vi "Settings.vi"() -> ()   [LabVIEW 2023]
uses:
  <vilib>/userDefined/High Color/nirio_resource_hc.ctl
panel:
  in  "?":T1(tab)
  in  "Current follower 1\n (AI-3)":dbl(ring)=-1e-08 items=["Raw"=1.0, "1mA (Ivium Compactstat.h)"=-0.001, "100uA (ivium Compactstat.h)"=-0.0001, "1uA (Ivium Compactstat.h)"=-1e-06, "100nA (Ivium Compactstat.h)"=-1e-07, "10nA (Ivium Compactstat.h)"=-1e-08, "1nA (Ivium Compactstat.h)"=-1e-09, "100pA (Ivium Compactstat.h)"=-1e-10, "10pA (Ivium Compactstat.h)"=-1e-11, "100 uA/V"=0.0001, "10 uA/V"=1e-05, "1 uA/V"=1e-06, "100 nA/V"=1e-07, "10 nA/V (0.1 mV/pA)"=1e-08, "0.2 mV/pA"=5e-09, "0.5 mV/pA"=2e-09, "1 nA/V (1 mV/pA)"=1e-09, "2 mV/pA"=5e-10, "5 mV/pA"=2e-10, "100 pA/V (10 mV/pA)"=1e-10, "20 mV/pA"=5e-11, "10 pA/V"=1e-11, "1 pA/V"=1e-12, "100 fA/V"=1e-13, "10 fA/V"=1e-14, "1 fA/V"=1e-15]
  in  "Current follower 3\n(AI-6)":dbl(ring)=1e-09 items=["Raw"=1.0, "100 uA/V"=0.0001, "10 uA/V"=1e-05, "1 uA/V"=1e-06, "100 nA/V"=1e-07, "10 nA/V (0.1 mV/pA)"=1e-08, "0.2 mV/pA"=5e-09, "0.5 mV/pA"=2e-09, "1 nA/V (1 mV/pA)"=1e-09, "2 mV/pA"=5e-10, "5 mV/pA"=2e-10, "100 pA/V (10 mV/pA)"=1e-10, "20 mV/pA"=5e-11, "10 pA/V"=1e-11, "1 pA/V"=1e-12, "100 fA/V"=1e-13, "10 fA/V"=1e-14, "1 fA/V"=1e-15]
  in  "Current follower 2 \n(AI-4)":dbl(ring)=-1.0 items=["Raw (Ivium Compactstat.h)"=-1.0, "10uA (Ivium Compactstat.h)"=-1e-05, "1uA (Ivium Compactstat.h)"=-1e-06, "100nA (Ivium Compactstat.h)"=-1e-07, "10nA (Ivium Compactsta.h)"=-1e-08, "1nA (Ivium Compactstat.h)"=-1e-09, "100pA (Ivium Compactstat.h)"=-1e-10, "10pA (Ivium Compactstat.h)"=-1e-11, "Raw"=1.0, "100 uA/V"=0.0001, "10 uA/V"=1e-05, "1 uA/V"=1e-06, "100 nA/V"=1e-07, "10 nA/V (0.1 mV/pA)"=1e-08, "0.2 mV/pA"=5e-09, "0.5 mV/pA"=2e-09, "1 nA/V (1 mV/pA)"=1e-09, "2 mV/pA"=5e-10, "5 mV/pA"=2e-10, "100 pA/V (10 mV/pA)"=1e-10, "20 mV/pA"=5e-11, "10 pA/V"=1e-11, "1 pA/V"=1e-12, "100 fA/V"=1e-13, "10 fA/V"=1e-14, "1 fA/V"=1e-15]
  in  "Lock In Sensitivity":dbl(ring)=1.0 items=["1V/V"=1.0, "500mV/V"=0.5, "200mV/V"=0.2]
  in  "Expand":dbl(ring)=100.0 items=["100"=100.0, "10"=10.0, "1"=1.0]
  in  "Percentage Offset":dbl min=0.0 max=100.0 step=0.0001 format="%#.12e"
  in  "Current follower for AC?":u8(ring) items=["C1", "C2", "C3"]
  in  "Sample Time (µs)":u32=4 min=2
  in  "Samples per Data Point":u16(ring)=512 items=["1"=1, "2"=2, "4"=4, "8"=8, "16"=16, "32"=32, "64"=64, "128"=128, "256"=256, "512"=512, "1024"=1024, "2048"=2048, "4096"=4096, "8192"=8192]
  in  "Save Folder Path":path=path "Z:/"
  in  "TempFilePath":path=path "C:/GitHub/WEC-SPM_Temp/test.tdms"
  in  "channel names":string[](array[string])=["X (um)", "Y (um)", "Z (um)", "V1 (V)", "V2 (V)", "Current1 (A)", "Current 2 (A)", "Current 3 (A)", "FeedbackType ", "Line Number", "Lockin Amplitude", "Lockin  Phase", "dt(s)"]
  in  "FPGA Target Device":T2="RIO0" caption="RIO Device"
  in  "Command Voltage2 Ratio 2":dbl(ring)=5.0 items=["1:1"=1.0, "5:1"=5.0, "10:1"=10.0]
  in  "Z piezo maximum range (µm)":dbl=200.0
  in  "Y piezo maximum range (µm)":dbl=200.0
  in  "X piezo maximum range (µm)":dbl=200.0
  in  "Command Voltage Ratio":dbl(ring)=1.0 items=["1:1"=1.0, "5:1"=5.0, "10:1"=10.0]
  out "Z (-10 to 10V)":bool
  out "X (-10 to 10V)":bool
  out "Y (-10 to 10V)":bool
  out "FPGA Speed [Hz]":i64=40000000
  in  "Host Path":path=path "C:/GitHub/WEC-SPM/Sub_Vi/FPGA/USB7855R_Specific/FPGA_Host_USB7855R.vi"
  out "Host To FPGA FIFO Length":i64=8196
  out "FIFO I16 per WayPoint":i64=15
  out "FIFO I16 per Sample":u32=14
  out "FPGA VI Reference":refnum<k20>
  in  "Points to Average":u16(ring)=1024 items=["1"=1, "2"=2, "4"=4, "8"=8, "16"=16, "32"=32, "64"=64, "128"=128, "256"=256, "512"=512, "1024"=1024, "2048"=2048, "4096"=4096, "8192"=8192]
  out "Waypoints per hop":dbl=3.0
  in  "Picomotor ScaleFactor":dbl=0.5
  out "FPGA \nrunning":bool
  out "Line Number":u64=1
  out "V2 (V)":dbl
  out "V (V)":dbl
  out "Z (µm)":dbl
  out "Y (µm)":dbl
  out "X (µm)":dbl
  # "Indicators"
  # "Current Follower Settings"
  # "External Lock In Settings"
  # "Save Settings"
  # "Data Collection Settings"
  # "Note: At high data collection rates (above 66 µs (2 µs, 32 points)) the computer may not be fast enough to collect the data, try disabling all plotting."
  # "Piezo Settings"
  # "FPGA Settings"
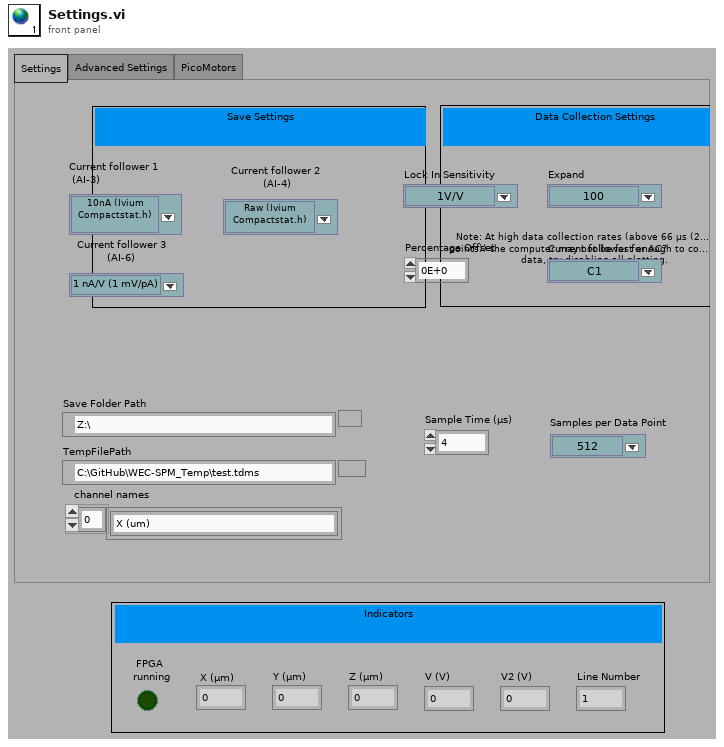
[diagram p1: front panel]
types:
  T1 = enum32{"Settings", "Advanced Settings", "PicoMotors"}
  T2 = typedef "nirio_resource_hc.ctl" = tag
diagram:
